vi "Retrieve_latest_PAQ_data.vi"(8 "error in (no error)":errorcluster, 10 "FetchLatestDefinition":T1, 11 "DBAL in":refnum<class "DBAL.lvclass">) -> (0 "error out":errorcluster, 2 "BinHistData":T2, 3 "DBAL out":refnum<class "DBAL.lvclass">)   [LabVIEW 2020, in "Sgraph_lib_V1.lvlib" / "DBAL.lvclass"]
uses:
  DBAL.lvclass
  controls/BIN/BINdata.ctl
  controls/DBAL_FetchLatestFrom.ctl
  DBAL-BIN.lvclass
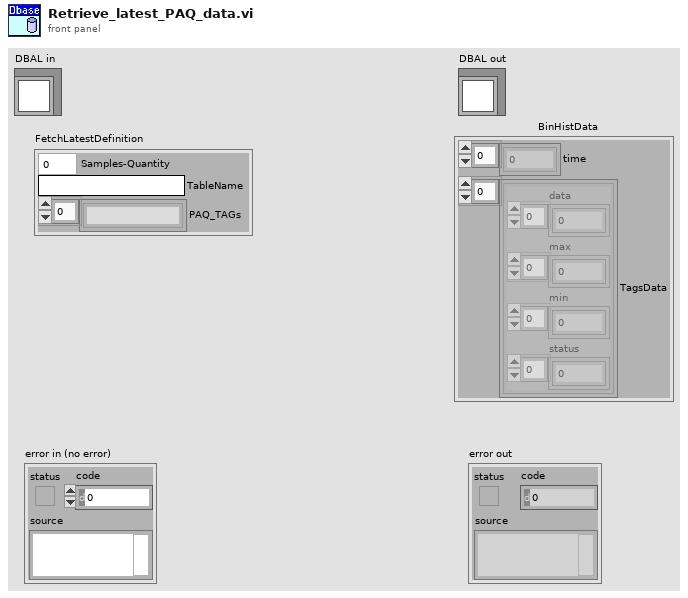
[diagram p1: front panel]
types:
  T1 = typedef "Sgraph_lib_V1.lvlib/DBAL.lvclass/DBAL_FetchLatestFrom.ctl" = cluster{"Samples-Quantity":i32, "TableName":string, "PAQ_TAGs":string[]}
  T2 = typedef "Sgraph_lib_V1.lvlib/DBAL-BIN.lvclass/BINdata.ctl" = cluster{"time":dbl[], "TagsData":cluster{"data":dbl[], "max":dbl[], "min":dbl[], "status":u32[]}[]}
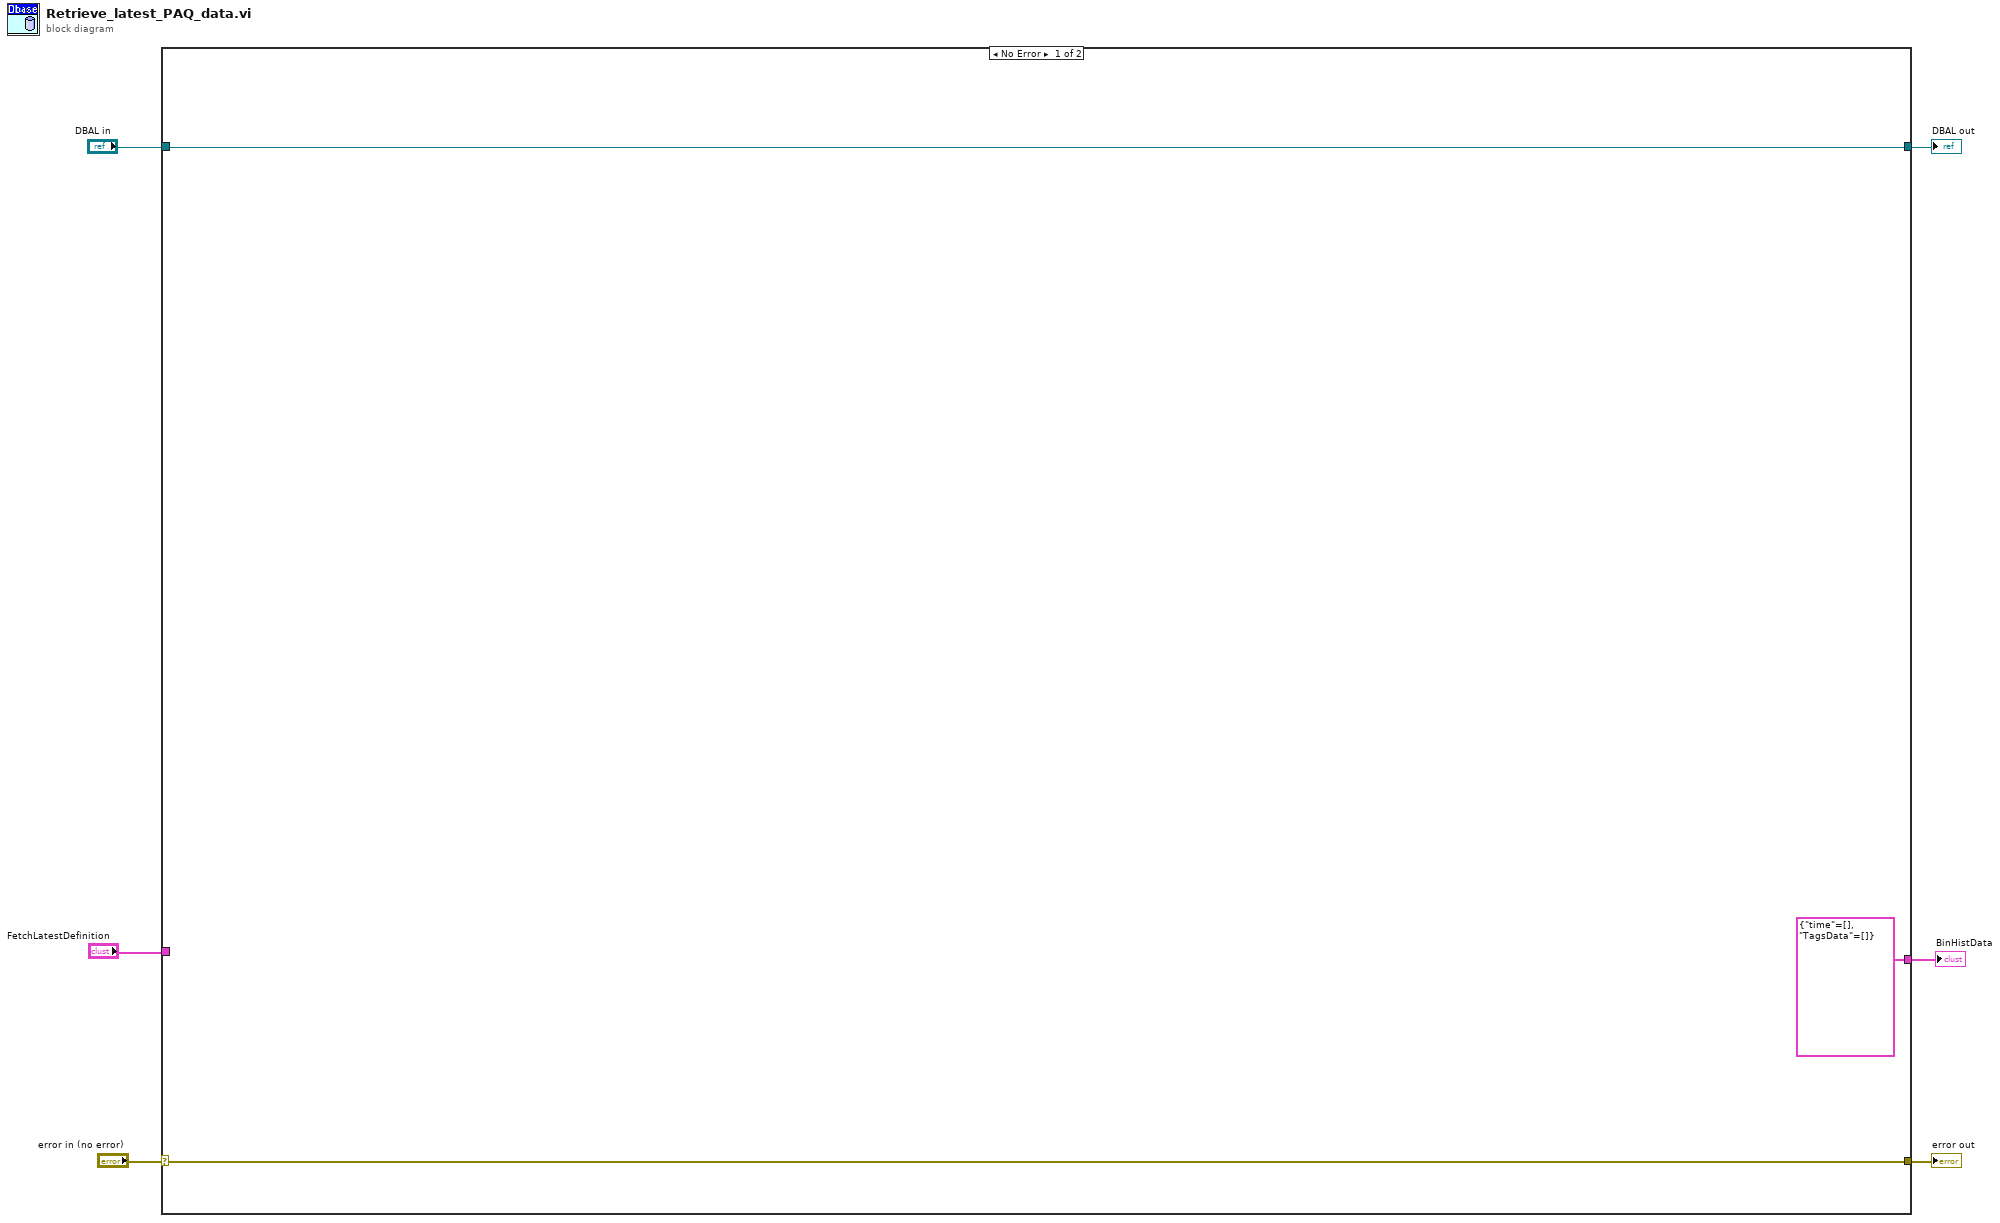
[diagram p0: block diagram]
diagram:
  n1 = case shown="No Error" "error in (no error)" {
    selector: "error in (no error)" -> [w9 w11]
    tunnel: [w9 w11] -> w5
    tunnel: [w7 w10] -> w4
    tunnel: "DBAL in" -> [w7 w10]
    tunnel: [T2 {"time"=[], "TagsData"=[]} ("BinHistData") _] -> w3
    tunnel: "FetchLatestDefinition" -> [_ _]
    frame No Error {
    }
    frame Error {
    }
  }
  "error out" <- w5
  "DBAL out" <- w4
  "BinHistData" <- w3
